vi "callUI.vi"(8 "Error In":errorcluster, 10 "UI Data":T1, 11 "UDE Data":T14) -> (0 "Error Out":errorcluster)   [LabVIEW 2018]
uses:
  UI Module/src/controls/uiUDE.ctl
  UI Module/src/controls/uiData.ctl
  controls/pathCluster.ctl
  UI Module/src/controls/shiftCluster.ctl
  UI Module/src/controls/modelHomeCluster.ctl
  UI Module/src/controls/hardwareSignalCluster.ctl
  UI Module/src/controls/printedBarcodeCluster.ctl
  UI Module/src/controls/scannedBarcode.ctl
  UI Module/src/controls/reportCluster.ctl
  UI Module/src/controls/modelSettingsCluster.ctl
  UI Module/src/controls/LHndRH.ctl
  UI Module/src/controls/ModelTableCluster.ctl
  UI Module/src/controls/overrideCluster.ctl
  UI Module/src/controls/countCluster.ctl
  controls/controllerData.ctl
  UI Module/src/controls/mainAppElementsCluster.ctl
  Modbus Module/src/controls/modbusData.ctl
  controls/readRegisterModbusCluster.ctl
  Barcode Printer Module/src/controls/printData.ctl
  Barcode Scanner Module/src/controls/scanData.ctl
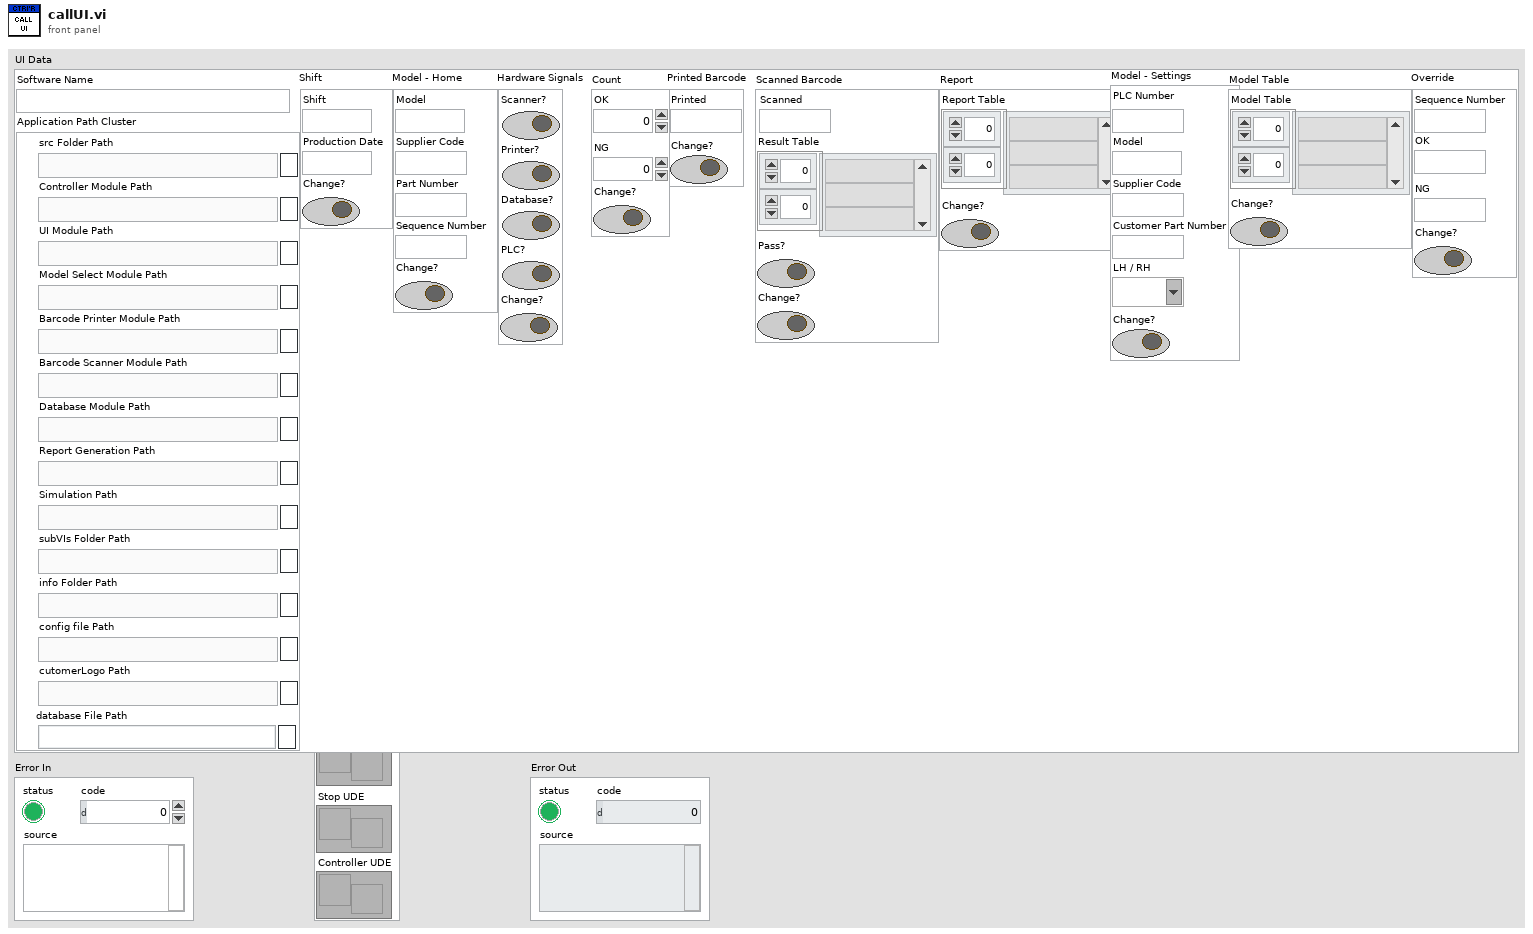
[diagram p1: front panel]
types:
  T1 = typedef "uiData.ctl" = cluster{"Software Name":string, "Application Path Cluster":T2, "Shift":T3, "Model - Home":T4, "Hardware Signals":T5, "Printed Barcode":T6, "Scanned Barcode":T7, "Report":T8, "Model - Settings":T9, "Model Table":T11, "Override":T12, "Count":T13}
  T2 = typedef "pathCluster.ctl" = cluster{"src Folder Path":path, "Controller Module Path":path, "UI Module Path":path, "Model Select Module Path":path, "Barcode Printer Module Path":path, "Barcode Scanner Module Path":path, "Database Module Path":path, "Report Generation Path":path, "Simulation Path":path, "subVIs Folder Path":path, "info Folder Path":path, "config file Path":path, "cutomerLogo Path":path, "database File Path":path}
  T3 = typedef "shiftCluster.ctl" = cluster{"Production Date":string, "Shift":string, "Change?":bool}
  T4 = typedef "modelHomeCluster.ctl" = cluster{"Model":string, "Supplier Code":string, "Part Number":string, "Sequence Number":string, "Change?":bool}
  T5 = typedef "hardwareSignalCluster.ctl" = cluster{"PLC?":bool, "Database?":bool, "Printer?":bool, "Scanner?":bool, "Change?":bool}
  T6 = typedef "printedBarcodeCluster.ctl" = cluster{"Printed":string, "Change?":bool}
  T7 = typedef "scannedBarcode.ctl" = cluster{"Scanned":string, "Result Table":string[][], "Change?":bool, "Pass?":bool}
  T8 = typedef "reportCluster.ctl" = cluster{"Report Table":string[][], "Change?":bool}
  T9 = typedef "modelSettingsCluster.ctl" = cluster{"Model":string, "Supplier Code":string, "Customer Part Number":string, "LH / RH":T10, "Change?":bool, "PLC Number":string}
  T10 = typedef "LHndRH.ctl" = string
  T11 = typedef "ModelTableCluster.ctl" = cluster{"Model Table":string[][], "Change?":bool}
  T12 = typedef "overrideCluster.ctl" = cluster{"Change?":bool, "Sequence Number":string, "OK":string, "NG":string}
  T13 = typedef "countCluster.ctl" = cluster{"Change?":bool, "OK":dbl, "NG":dbl}
  T14 = typedef "uiUDE.ctl" = cluster{"UI UDE":refnum<user-event>, "Stop UDE":refnum<user-event>, "Controller UDE":refnum<user-event>}
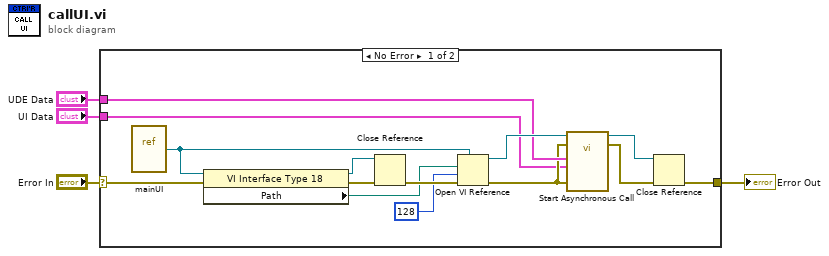
[diagram p0: block diagram]
diagram:
  n1 = case shown="No Error" "Error In" {
    selector: "Error In" -> [w18 w19]
    tunnel: [w9 w19] -> w3
    tunnel: "UDE Data" -> [w7 _]
    tunnel: "UI Data" -> [w5 _]
    frame No Error {
      n2 = vi-ref "mainUI.vi"() -> (w11:refnum<vi>)
      n3 = property class="VI Interface Type 18"(reference=w11, error in=w18) -> (reference out=w16:refnum<vi>, error out=w17:errorcluster, "Path"=w14:path)
      n4 = Close Reference(reference=w16, error in (no error)=w17) -> (error out=w15:errorcluster)
      n5 = Open VI Reference(type specifier VI Refnum (for type only)=w11, vi path=w14, options=128, error in (no error)=w15) -> (vi reference=w12:refnum<vi>, error out=w6:errorcluster)  [unwired: 2 in]
      n6 = call-by-ref "Start Asynchronous Call"(reference=w12, error in=w6, "Error In"=w6, "UI Data"=w5, "UDE Data"=w7) -> (reference out=w8:refnum<vi>, error out=w10:errorcluster)  [unwired: 8 in, 1 out]
      n7 = Close Reference(reference=w8, error in (no error)=w10) -> (error out=w9:errorcluster)
    }
    frame Error {
    }
  }
  "Error Out" <- w3
